vi "ParseJSON.vi"() -> ()   [LabVIEW 2019, in "SLL JSON to Cluster.lvlib"]
doc: "This VI converts a JSON string into its corresponding cluster type within the specified VI, if the provided path is valid. If the path is invalid or the VI doesn't exist, it creates a new VI and generates the cluster within it. also, If Update Values enabled, cluster will be updated with JSON data."
uses:
  SLL JSON to Cluster.lvlib
panel:
  in  "Update Values":bool
  out "Error Out":errorcluster
  in  "Error In":errorcluster
  in  "VI Path To Create Cluster":path
  in  "JSON String":string="{\n  \"office\": \"HQ Main Building\",\n  \"location\": \"New York City\",\n  \"clusters\": [\n    {\n      \"clusterId\": \"alpha-01\",\n      \"department\": \"Engineering\",\n      \"nodes\": [\n        {\"nodeId\": \"eng-001\", \"status\": \"active\", \"ip\": \"10.0.0.1\"},\n        {\"nodeId\": \"eng-002\", \"status\": \"active\", \"ip\": \"10.0.0.2\"},\n        {\"nodeId\": \"eng-003\", \"status\": \"inactive\", \"ip\": \"10.0.0.3\"}\n      ],\n      \"services\": [\"CI/CD\", \"Version Control\", \"Monitoring\"]\n    },\n    {\n      \"clusterId\": \"beta-02\",\n      \"department\": \"Marketing\",\n      \"nodes\": [\n        {\"nodeId\": \"mkt-101\", \"status\": \"active\", \"ip\": \"10.1.0.1\"},\n        {\"nodeId\": \"mkt-102\", \"status\": \"maintenance\", \"ip\": \"10.1.0.2\"}\n      ],\n      \"services\": [\"Email Campaigns\", \"Analytics\"]\n    },\n    {\n      \"clusterId\": \"gamma-03\",\n      \"department\": \"HR\",\n      \"nodes\": [\n        {\"nodeId\": \"hr-201\", \"status\": \"active\", \"ip\": \"10.2.0.1\"},\n        {\"nodeId\": \"hr-202\", \"status\": \"active\", \"ip\": \"10.2.0.2\"},\n        {\"nodeId\": \"hr-203\", \"status\": \"active\", \"ip\": \"10.2.0.3\"},\n        {\"nodeId\": \"hr-204\", \"status\": \"inactive\", \"ip\": \"10.2.0.4\"}\n      ],\n      \"services\": [\"Payroll\", \"Recruitment Portal\", \"Employee Records\"]\n    }\n  ]\n}\n"
  # "JSON To Cluster"
  # "Steps to Convert JSON to Cluster:\n1. Provide the input JSON string that you wish to convert into a cluster.\n2. Run the VI.\n3. The cluster will be created either in the specified VI path or in a new VI, if VI path is provided.\n4. If Update Values enabled, cluster will be updated with JSON data."
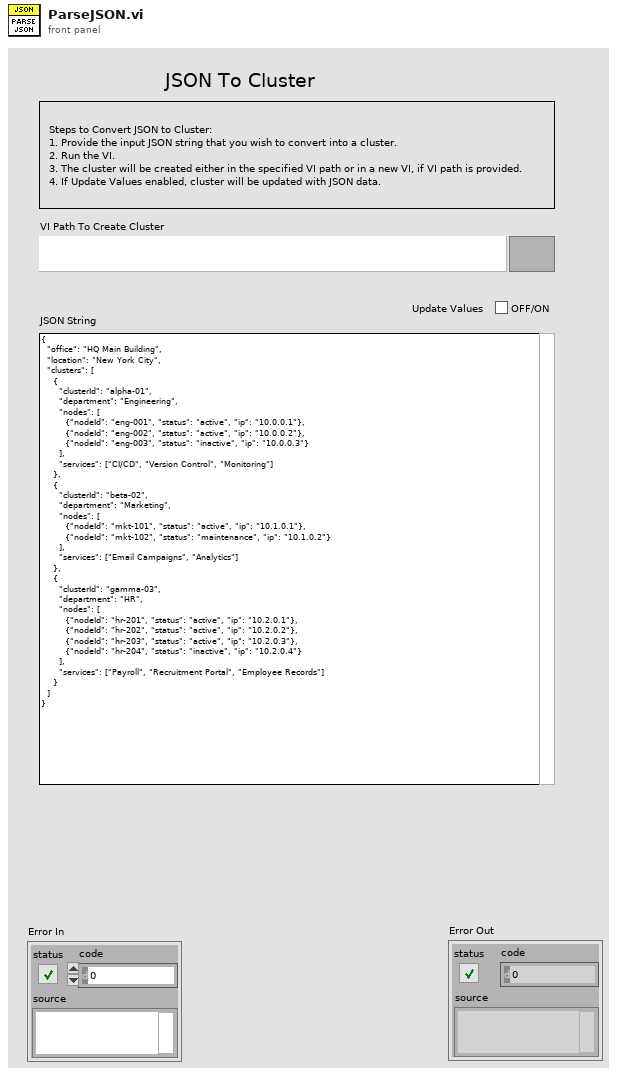
[diagram p1: front panel]
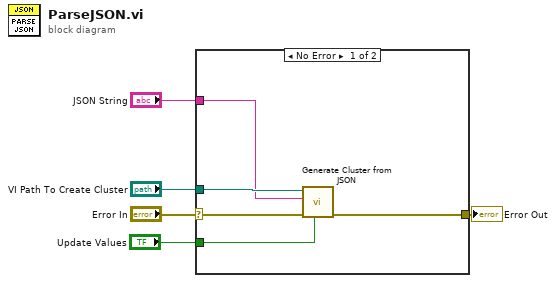
[diagram p0: block diagram]
diagram:
  n1 = case shown="No Error" "Error In" {
    selector: "Error In" -> [w10 w11]
    tunnel: "JSON String" -> [w8 _]
    tunnel: "VI Path To Create Cluster" -> [w9 _]
    tunnel: [w7 w11] -> w2
    tunnel: "Update Values" -> [w6 _]
    frame No Error {
      n2 = call "Generate Cluster from JSON.vi"("Update Values"=w6, "Error In"=w10, "JSON String"=w8, "VI Path"=w9) -> ("Errror Out"=w7:errorcluster)  [unwired: 7 in]
    }
    frame Error {
    }
  }
  "Error Out" <- w2
